vi "UTILITY Modbus 16bit Number Combine.vi"(11 "Holding Registers":u16[](array[numeric])) -> (3 "Data":dbl)   [LabVIEW 2016]
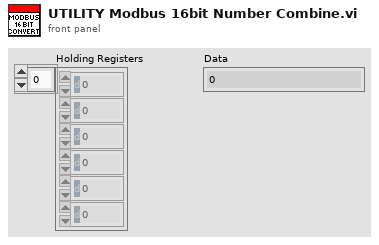
[diagram p1: front panel]
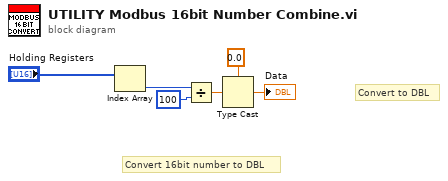
[diagram p0: block diagram]
diagram:
  # "Convert to DBL"
  # "Convert 16bit number to DBL"
  n1 = Index Array(array="Holding Registers") -> (element=w4:u16)  [unwired: 1 in]
  n2 = Divide(x=w4, y=u16 100) -> (x/y=w1:dbl)
  n3 = Type Cast(type=0.0, x=w1) -> (*(type *) &x=→"Data":dbl)
